vi "GetPosSingleAxis.vi"(8 "error in (no error)":errorcluster, 10 "Axis":i32=1 min=1 max=4, 11 "OWIS_TANGO in":refnum<class "OWIS_TANGO.lvclass">) -> (0 "error out":errorcluster, 2 "Pos":dbl, 3 "OWIS_TANGO out":refnum<class "OWIS_TANGO.lvclass">)   [LabVIEW 2020, in "OWIS_TANGO.lvclass"]
uses:
  OWIS_TANGO.lvclass
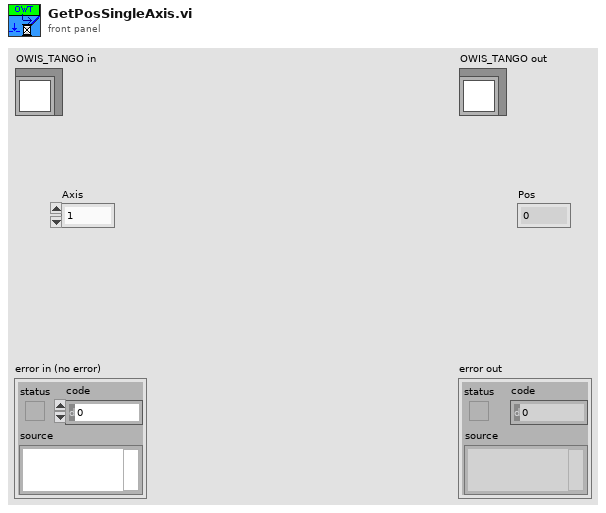
[diagram p1: front panel]
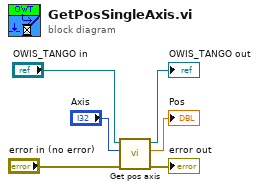
[diagram p0: block diagram]
diagram:
  n1 = call-dynamic "Get pos axis.vi"("error in (no error)"="error in (no error)", "Axis"="Axis", "OWIS_TANGO in"="OWIS_TANGO in") -> ("error out"=→"error out":errorcluster, "Pos"=→"Pos":dbl, "OWIS_TANGO out"=→"OWIS_TANGO out":refnum<class "OWIS_TANGO.lvclass">)  [unwired: 6 in]
